vi "createScan.vi"(8 "error in (no error)":errorcluster, 10 "delayAll":bool, 11 "ScanCreator in":refnum<class "ScanCreator.lvclass">) -> (0 "error out":errorcluster, 1 "scriptListArray":refnum<class "ScriptEventList.lvclass">[](array[class]), 2 "close":bool, 3 "ScanCreator out":refnum<class "ScanCreator.lvclass">, 4 "scanType":string, 5 "Values":string[](array[string]))   [LabVIEW 2009, in "Views.lvlib" / "ScriptEditor.lvlib" / "ScanCreator.lvclass"]
uses:
  ScanCreator.lvclass
  Tools/Scripting/ScriptingEvent/ScriptEventList/ScriptEventList.lvclass
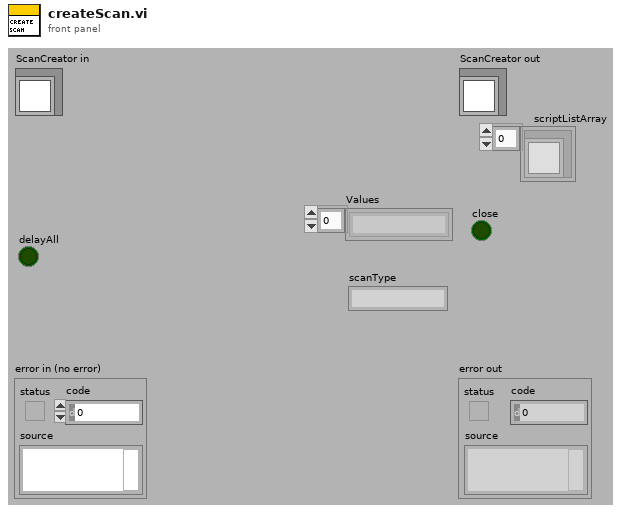
[diagram p1: front panel]
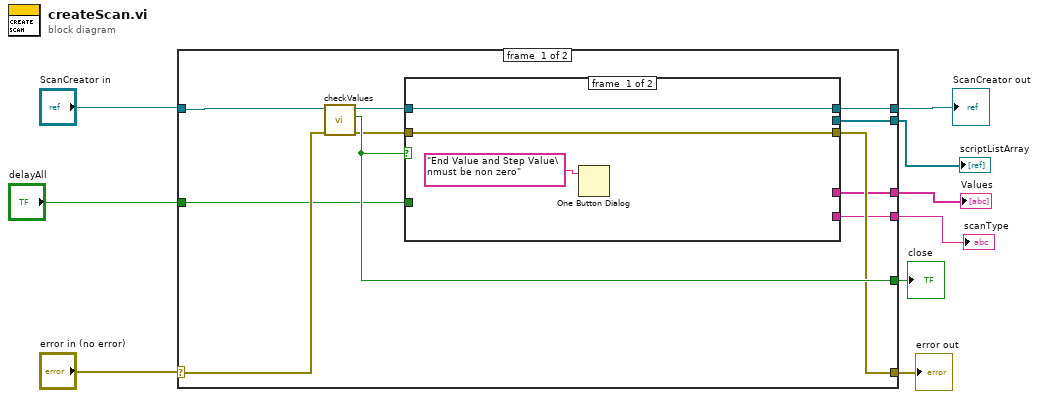
[diagram p0: block diagram]
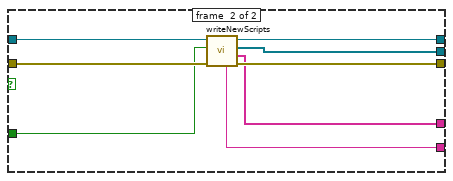
[diagram p2: hidden frame]
diagram:
  n1 = case shown="No Error" "error in (no error)" {
    selector: "error in (no error)" -> [w20 w33]
    tunnel: [w15 w33] -> w8
    tunnel: [w16 w32] -> w6
    tunnel: "ScanCreator in" -> [w14 w32]
    tunnel: [w18 _] -> w5
    tunnel: "delayAll" -> [w13 _]
    tunnel: [w12 _] -> w3
    tunnel: [w11 _] -> w2
    tunnel: [w10 _] -> w1
    frame #0 {
      n2 = call "checkValues.vi"("error in (no error)"=w20, "ScanCreator in"=w14) -> ("error out"=w17:errorcluster, "passed"=w18:bool, "ScanCreator out"=w19:refnum<class "ScanCreator.lvclass">)  [unwired: 7 in]
      n3 = case shown="True" w18 {
        tunnel: w19 -> [w22 w31]
        tunnel: w17 -> [w21 w29]
        tunnel: [w22 w30] -> w16
        tunnel: [w21 w28] -> w15
        tunnel: w13 -> [_ w27]
        tunnel: [_ w26] -> w12
        tunnel: [_ w25] -> w11
        tunnel: [_ w24] -> w10
        frame #0 {
          n4 = One Button Dialog(message="End Value and Step Value\nmust be non zero") -> ()  [unwired: 1 in, 1 out]
        }
        frame #1 {
          n5 = call "writeNewScripts.vi"("error in (no error)"=w29, "delayAll"=w27, "ScanCreator in"=w31) -> ("error out"=w28:errorcluster, "Values"=w25:string[], "scriptListArray"=w26:refnum<class "ScriptEventList.lvclass">[], "ScanCreator out"=w30:refnum<class "ScanCreator.lvclass">, "scanType"=w24:string)  [unwired: 4 in]
        }
      }
    }
    frame #1 {
    }
  }
  "error out" <- w8
  "ScanCreator out" <- w6
  "close" <- w5
  "scriptListArray" <- w3
  "Values" <- w2
  "scanType" <- w1
